vi "CheckStreamConnection.vi"(8 "error in":errorcluster, 11 "ref":refnum<k21>) -> (0 "error out":errorcluster, 2 "Connected":bool, 3 "ref":refnum<k21>)   [LabVIEW 2018]
uses:
  RT/Queue/RTMainQueueElements.ctl
  <resource>/objmgr/ni.dex.rc
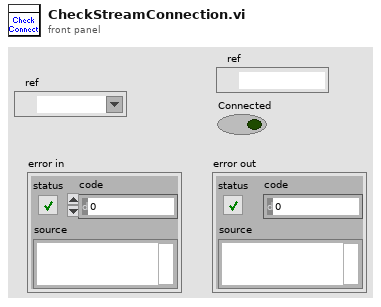
[diagram p1: front panel]
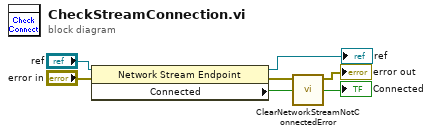
[diagram p0: block diagram]
diagram:
  n1 = property class="Network Stream Endpoint"(reference="ref", error in="error in") -> (reference out=→"ref":refnum<k21>, error out=w4:errorcluster, "Connected"=→"Connected":bool)
  n2 = call "ClearNetworkStreamNotConnectedError.vi"("ErrorIn"=w4) -> ("ErrorOut"=→"error out":errorcluster)  [unwired: 10 in]
